vi "Initialize Camera and CheckList.vi"(11 "ListBox in":refnum<vi>) -> ()   [LabVIEW 2020]
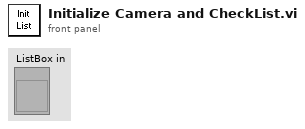
[diagram p1: front panel]
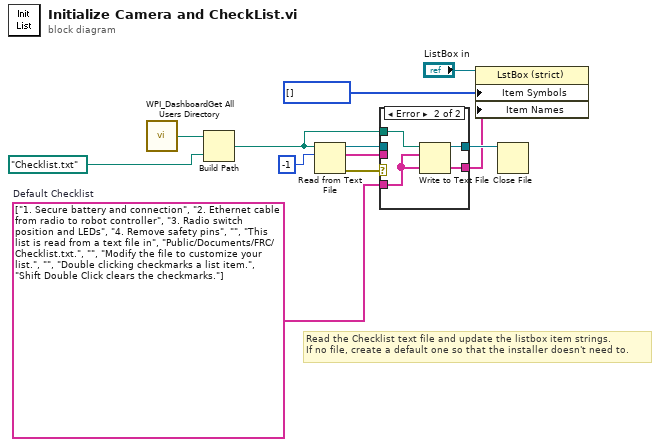
[diagram p0: block diagram]
diagram:
  w9 = string[] ["1. Secure battery and connection", "2. Ethernet cable from radio to robot controller", "3. Radio switch position and LEDs", "4. Remove safety pins", "", "This list is read from a text file in", "Public/Documents/FRC/Checklist.txt.", "", "Modify the file to customize your list.", "", "Double clicking checkmarks a list item.", "Shift Double Click clears the checkmarks."]  # Default Checklist
  # "Read the Checklist text file and update the listbox item strings.\nIf no file, create a default one so that the installer doesn't need to."
  n1 = call <vilib>:"WPI_DashboardGet All Users Directory.vi"() -> ("All User Path"=w10:path)
  n2 = Build Path(base path=w10, name or relative path=path "Checklist.txt") -> (appended path=w1:path)
  n3 = Read from Text File(file (use dialog)=w1, count=-1 ("timeout ms (25000)")) -> (refnum out=w11:refnum<file>, text=w8:string[], error out=w7:errorcluster)  [unwired: 2 in, 1 out]
  n4 = case shown="Error" w7 {
    tunnel: w8 -> [w14 _]
    tunnel: [w14 w16] -> w2
    tunnel: w9 -> [_ w16]
    tunnel: w1 -> [_ w17]
    tunnel: [w13 w15] -> w12
    tunnel: w11 -> [w13 _]
    frame No Error {
    }
    frame Error {
      n5 = Write to Text File(file (use dialog)=w17, text=w16) -> (refnum out=w15:refnum<file>)  [unwired: 2 in, 2 out]
    }
  }
  n6 = property on="Property Node" class="LstBox (strict)"(reference="ListBox in", "Item Symbols"=i32[] [], "Item Names"=w2) -> ()  [unwired: 1 in, 2 out]
  n7 = Close File(refnum=w12) -> ()  [unwired: 1 in, 2 out]
